vi "levelrefilltest.vi"() -> ()   [LabVIEW 2023]
uses:
  AutomatedSetupAcousticEnergyDensity/CetoniPump_class/CetoniPump.lvclass
  Application_class/Application.lvclass
panel:
  in  "Timeout Refill":dbl=20.0 caption="Time Target (s)"
  in  "refill below level":dbl
  in  "index":i32
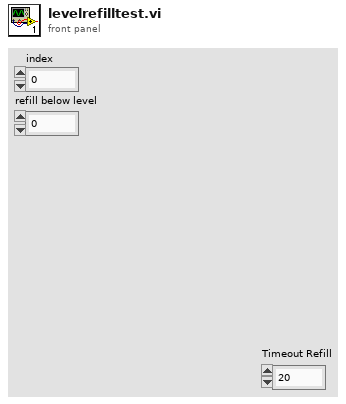
[diagram p1: front panel]
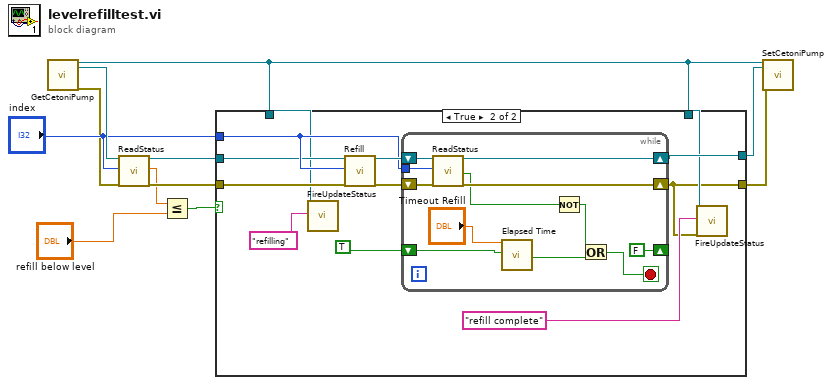
[diagram p0: block diagram]
diagram:
  n1 = call-dynamic "GetCetoniPump.vi"() -> ("object in"=w14:refnum<class "Application.lvclass">, "error in (no error)"=w12:errorcluster, "object out"=w1:refnum<class "Application.lvclass">, "CetoniPump"=w11:refnum<class "CetoniPump.lvclass">, "error out"=w3:errorcluster)  [unwired: 15 in]
  n2 = call-dynamic "ReadStatus.vi"("object in"=w11, "index"="index", "error in (no error)"=w3) -> ("object out"=w9:refnum<class "CetoniPump.lvclass">, "Fill Level"=w6:dbl, "error out"=w8:errorcluster)  [unwired: 12 in, 2 out]
  n3 = Less Or Equal?(x=w6, y="refill below level") -> (x <= y?=w7:bool)
  n4 = case shown="True" w7 {
    tunnel: "index" -> [_ w27]
    tunnel: w9 -> [w16 w23]
    tunnel: w8 -> [w15 w25]
    tunnel: [w16 w20] -> w4
    tunnel: [w15 w17] -> w2
    tunnel: w1 -> [_ w22]
    tunnel: w1 -> [_ w19]
    frame False {
    }
    frame True {
      n5 = call-dynamic "FireUpdateStatus.vi"("object in"=w22, "Status"="refilling") -> ()  [unwired: 16 in, 2 out]
      n6 = call-dynamic "Refill.vi"("object in"=w23, "index"=w27, "error in (no error)"=w25) -> ("object out"=w28:refnum<class "CetoniPump.lvclass">, "error out"=w26:errorcluster)  [unwired: 15 in]
      n7 = while {
        tunnel: w27 -> [w39]
        shift-right: [w29] -> w20
        shift-left: w28 -> [w40]
        shift-right: [w37] -> w17
        shift-left: w26 -> [w38]
        shift-right: [FALSE] -> _
        shift-left: TRUE -> [w31]
        stop <- w32 stop-if-true
        n8 = call-dynamic "ReadStatus.vi"("object in"=w40, "index"=w39, "error in (no error)"=w38) -> ("object out"=w29:refnum<class "CetoniPump.lvclass">, "Is pumping"=w35:bool, "error out"=w37:errorcluster)  [unwired: 12 in, 2 out]
        n9 = call "Elapsed Time"("Time Target (s)"="Timeout Refill", "Reset"=w31) -> ("Time has Elapsed"=w33:bool)  [unwired: 10 in, 7 out]
        n10 = Not(x=w35) -> (.not. x?=w34:bool)
        n11 = Or(x=w34, y=w33) -> (x .or. y?=w32:bool)
      }
      n12 = call-dynamic "FireUpdateStatus.vi"("object in"=w19, "Status"="refill complete", "error in (no error)"=w17) -> ()  [unwired: 15 in, 2 out]
    }
  }
  n13 = call-dynamic "SetCetoniPump.vi"("object in"=w1, "CetoniPump"=w4, "error in (no error)"=w2) -> ("error out"=w13:errorcluster)  [unwired: 15 in, 1 out]
